vi "Clear_Info.vi"(8 "error in (no error)":errorcluster, 9 "index in":string, 10 "buildObject":T1) -> (0 "error out":errorcluster, 1 "index out":string, 2 "buildObject out":T1)   [LabVIEW 2020, in "IB_RegDest.lvclass"]
uses:
  <vilib>/AppBuilder/IB_Classes/RegDest/IB_RegDest.lvclass
  <vilib>/AppBuilder/IB_Classes/RegDest/IB_RegDest.lvclass/IB_RegDest.ctl
  <vilib>/AppBuilder/IB_RW_Project/IB_RW_Project_PropBag_Action.ctl
  <resource>/Framework/Providers/API/ItemRef.ctl
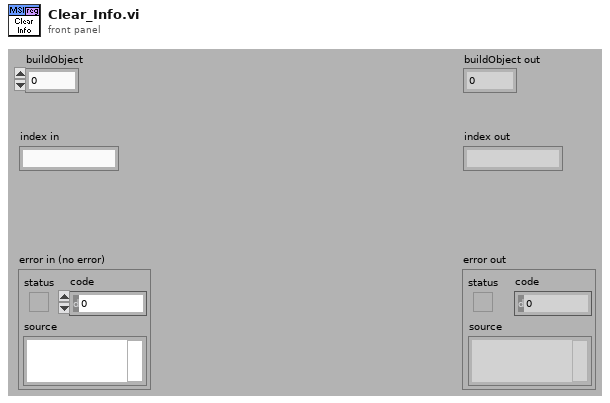
[diagram p1: front panel]
types:
  T1 = typedef "ItemRef.ctl" = u64
  T2 = typedef "IB_RW_Project_PropBag_Action.ctl" = enum16{"read", "write", "clear", "readPrevious", "writePrevious", "clearPrevious"}
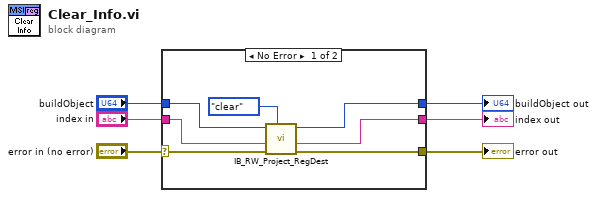
[diagram p0: block diagram]
diagram:
  n1 = case shown="No Error" "error in (no error)" {
    selector: "error in (no error)" -> [w12 w16]
    tunnel: [w11 w16] -> w5
    tunnel: "buildObject" -> [w9 w15]
    tunnel: [w8 w15] -> w3
    tunnel: "index in" -> [w10 w14]
    tunnel: [w7 w14] -> w1
    frame No Error {
      n2 = call <vilib>:"IB_RW_Project_RegDest.vi"("action"=IB_RW_Project_PropBag_Action."clear", "error in (no error)"=w12, "index in"=w10, "buildObject"=w9) -> ("error out"=w11:errorcluster, "index out"=w7:string, "buildObject out"=w8:T1)  [unwired: 4 in, 1 out]
    }
    frame Error {
    }
  }
  "error out" <- w5
  "index out" <- w1
  "buildObject out" <- w3
